vi "Complement with Fixed Parameters.vi"(8 "Fit Model":T2, 9 "Fixed Parameter Values":dbl[](array[numeric]), 10 "Fitted Parameter Names":T1[](array[typedef]), 11 "Fitted parameters (with sigma) in":dbl[](array[numeric])) -> (3 "Fitted parameters (with sigma) out":dbl[](array[numeric]))   [LabVIEW 2021, in "Fits.lvlib"]
doc: "Merges fitted and fixed parameters of a n-Exp fit into an ordered list."
uses:
  Fits.lvlib
  Decay Model.ctl
  IRF(X)PSED/Decay Fit Parameters In List.ctl
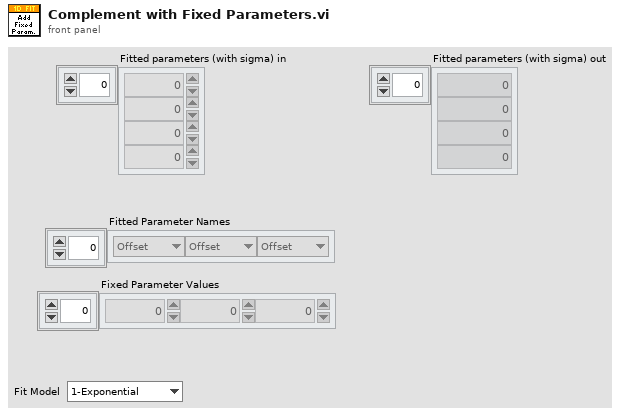
[diagram p1: front panel]
types:
  T1 = typedef "Fits.lvlib/Decay Fit Parameters In List.ctl" = enum16{"Offset", "Baseline", "A_1", "tau_1", "A_2", "tau_2"}
  T2 = typedef "Fits.lvlib/Decay Model.ctl" = enum16{"1-Exponential", "2-Exponentials"}
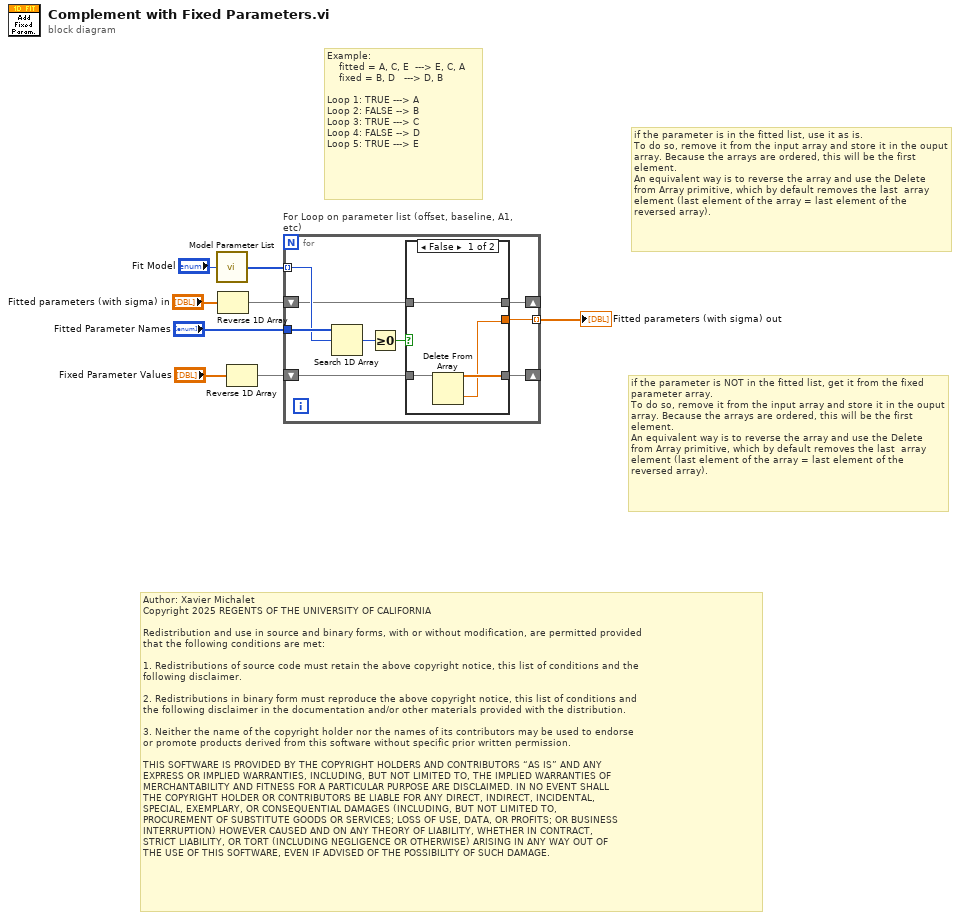
[diagram p0: block diagram]
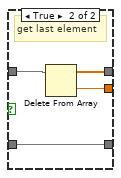
[diagram p2: hidden frame]
diagram:
  # "if the parameter is NOT in the fitted list, get it from the fixed parameter array.\nTo do so, remove it from the input array and store it in the ouput array. Because the arrays are ordered, this will be the first element.\nAn equivalent way is to reverse the array and use the Delete from Array primitive, which by default removes the last  array element (last element of the array = last element of the reversed array)."
  # "if the parameter is in the fitted list, use it as is.\nTo do so, remove it from the input array and store it in the ouput array. Because the arrays are ordered, this will be the first element.\nAn equivalent way is to reverse the array and use the Delete from Array primitive, which by default removes the last  array element (last element of the array = last element of the reversed array)."
  # "Author: Xavier Michalet\nCopyright 2025 REGENTS OF THE UNIVERSITY OF CALIFORNIA\n\nRedistribution and use in source and binary forms, with or without modification, are permitted provided\nthat the following conditions are met:\n\n1. Redistributions of source code must retain the above copyright notice, this list of conditions and the\nfollowing disclaimer.\n\n2. Redistributions in binary form must reproduce the above copyright notice, this list of conditions and\nthe following disclaimer in the documentation and/or other materials provided with the distribution.\n\n3. Neither the name of the copyright holder nor the names of its contributors may be used to endorse \nor promote products derived from this software without specific prior written permission.\n\nTHIS SOFTWARE IS PROVIDED BY THE COPYRIGHT HOLDERS AND CONTRIBUTORS “AS IS” AND ANY \nEXPRESS OR IMPLIED WARRANTIES, INCLUDING, BUT NOT LIMITED TO, THE IMPLIED WARRANTIES OF\nMERCHANTABILITY AND FITNESS FOR A PARTICULAR PURPOSE ARE DISCLAIMED. IN NO EVENT SHALL\nTHE COPYRIGHT HOLDER OR CONTRIBUTORS BE LIABLE FOR ANY DIRECT, INDIRECT, INCIDENTAL, \nSPECIAL, EXEMPLARY, OR CONSEQUENTIAL DAMAGES (INCLUDING, BUT NOT LIMITED TO, \nPROCUREMENT OF SUBSTITUTE GOODS OR SERVICES; LOSS OF USE, DATA, OR PROFITS; OR BUSINESS\nINTERRUPTION) HOWEVER CAUSED AND ON ANY THEORY OF LIABILITY, WHETHER IN CONTRACT, \nSTRICT LIABILITY, OR TORT (INCLUDING NEGLIGENCE OR OTHERWISE) ARISING IN ANY WAY OUT OF\nTHE USE OF THIS SOFTWARE, EVEN IF ADVISED OF THE POSSIBILITY OF SUCH DAMAGE."
  # "Example:\n    fitted = A, C, E  ---> E, C, A\n    fixed = B, D   ---> D, B\n\nLoop 1: TRUE ---> A\nLoop 2: FALSE --> B\nLoop 3: TRUE ---> C\nLoop 4: FALSE --> D\nLoop 5: TRUE ---> E"
  n1 = call "Model Parameter List.vi"("Fit Model"="Fit Model") -> ("Model Parameter List"=w7:T1[])
  n2 = Reverse 1D Array(array="Fitted parameters (with sigma) in") -> (reversed array=w4:dbl[])
  n3 = Reverse 1D Array(array="Fixed Parameter Values") -> (reversed array=w1:dbl[])
  n4 = for "For Loop on parameter list (offset, baseline, A1, etc)" {
    tunnel: w7 -> [w16] mode=indexing
    tunnel: "Fitted Parameter Names" -> [w17]
    shift-right: [w13] -> _
    shift-left: w4 -> [w14]
    tunnel: [w11] -> w3 mode=indexing
    shift-right: [w9] -> _
    shift-left: w1 -> [w10]
    n5 = Search 1D Array(1D array=w17, element=w16) -> (index of element=w15:i32)  [unwired: 1 in]
    n6 = Greater Or Equal To 0?(x=w15) -> (x >= 0?=w12:bool)
    n7 = case shown="False" w12 {
      tunnel: w14 -> [w21 w25]
      tunnel: [w21 w24] -> w13
      tunnel: [w18 w23] -> w11
      tunnel: w10 -> [w20 w22]
      tunnel: [w19 w22] -> w9
      frame False {
        n8 = Delete From Array(array=w20) -> (deleted portion=w18:dbl, array with subset deleted=w19:dbl[])  [unwired: 2 in]
      }
      frame True {
        # "get last element"
        n9 = Delete From Array(array=w25) -> (deleted portion=w23:dbl, array with subset deleted=w24:dbl[])  [unwired: 2 in]
      }
    }
  }
  "Fitted parameters (with sigma) out" <- w3
